vi "Get Progress by val.vi"(8 "error in (no error)":errorcluster, 11 "HTTP GET Async in":refnum<class "GET Async.lvclass">) -> (0 "error out":errorcluster, 1 "percent complete":dbl, 2 "bytes downloaded":i64, 3 "HTTP GET Async out":refnum<class "GET Async.lvclass">, 5 "file size":i64)   [LabVIEW 2019, in "HTTP Client Extensions.lvlib" / "GET Async.lvclass"]
uses:
  GET Async.lvclass
  GET Async.lvclass/GET Async.ctl
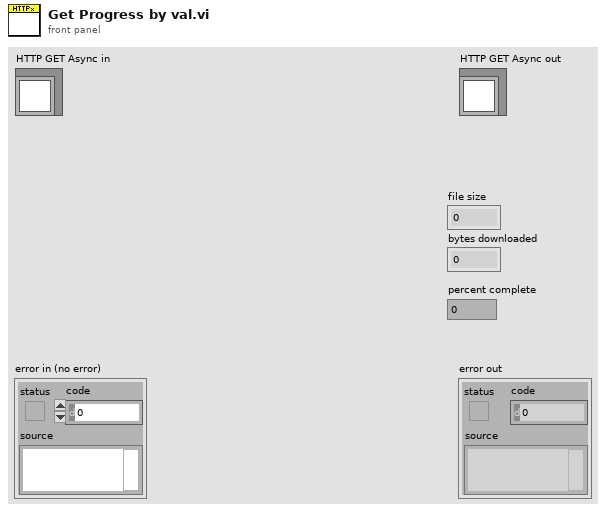
[diagram p1: front panel]
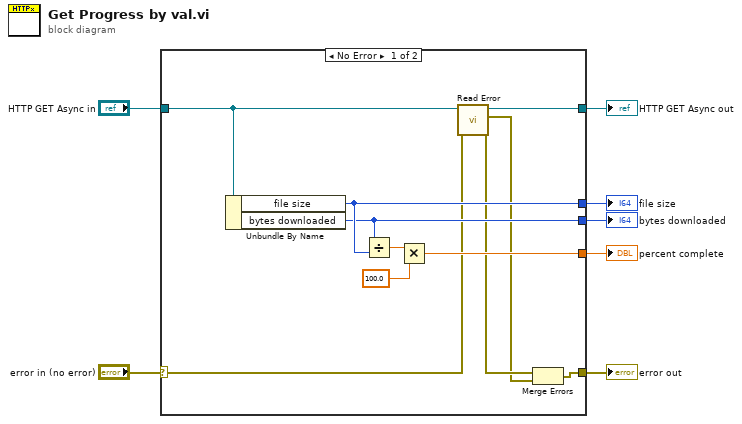
[diagram p0: block diagram]
diagram:
  n1 = case shown="No Error" "error in (no error)" {
    selector: "error in (no error)" -> [w11 w20]
    tunnel: [w9 w20] -> w6
    tunnel: [w13 w19] -> w4
    tunnel: "HTTP GET Async in" -> [w12 w19]
    tunnel: [w16 _] -> w3
    tunnel: [w15 _] -> w2
    tunnel: [w14 _] -> w1
    frame No Error {
      n2 = Unbundle By Name(w12) -> ("file size"=w16:i64, "bytes downloaded"=w15:i64)
      n3 = Divide(x=w15, y=w16) -> (x/y=w18:dbl)
      n4 = Multiply(x=w18, y=100.0) -> (x*y=w14:dbl)
      n5 = call "Read Error.vi"("error in (no error)"=w11, "GET Async in"=w12) -> ("error out"=w10:errorcluster, "error"=w8:errorcluster, "GET Async out"=w13:refnum<class "GET Async.lvclass">)  [unwired: 7 in]
      n6 = Merge Errors(w10, w8) -> (w9:errorcluster)
    }
    frame Error {
    }
  }
  "error out" <- w6
  "HTTP GET Async out" <- w4
  "file size" <- w3
  "bytes downloaded" <- w2
  "percent complete" <- w1
